vi "Reduce Vitrek Results.vi"(0 "Results String":string, 1 "BW1 ACW Time":string[](array[string]), 2 "BW1 ACW Raw":string[](array[string]), 3 "BW2 ACW Time":string[](array[string]), 4 "BW2 ACW Raw":string[](array[string]), 5 "error in (no error)":errorcluster, 6 "Result Error Status":string, 7 "Dielectric Strength Spec (uA)":dbl=50.0 format="%#_13g", 9 "Insulation Resistance Spec (Mohms)":dbl=100.0 format="%#_13g") -> (11 "BW1 Results Indicator":T1, 13 "BW2 Results Indicator":T1, 14 "Raw Data ACW BW1":T4, 15 "BW 1 Results":T2, 16 "Raw Data ACW BW2":T3, 17 "BW 2 Results":T2, 19 "error out":errorcluster)   [LabVIEW 2018]
panel:
  out "BW2 Insulation Resistance":string
  out "BW1 Insulation Resistance":string
  out "BW2 IR Pass Indicator":u16
  out "BW2 IR Pass?":bool
  out "BW1 IR Pass Indicator":u16
  out "BW1 IR Pass?":bool
  out "BW1 ACW Pass Indicator":u16
  out "BW1 Dielectric Strength Pass?":bool
  out "BW2 Dielectric Strength Pass?":bool
  out "BW2 Max Leakage Current":dbl
  out "BW2 Min Leakage Current":dbl
  out "BW1 Min Leakage Current":dbl
  out "BW1 Max Leakage Current":dbl
  out "BW2 ACW Pass Indicator":u16
  out "BW2 Max Change in Current (A)":dbl
  out "BW1 Max Change in Current (A)":dbl
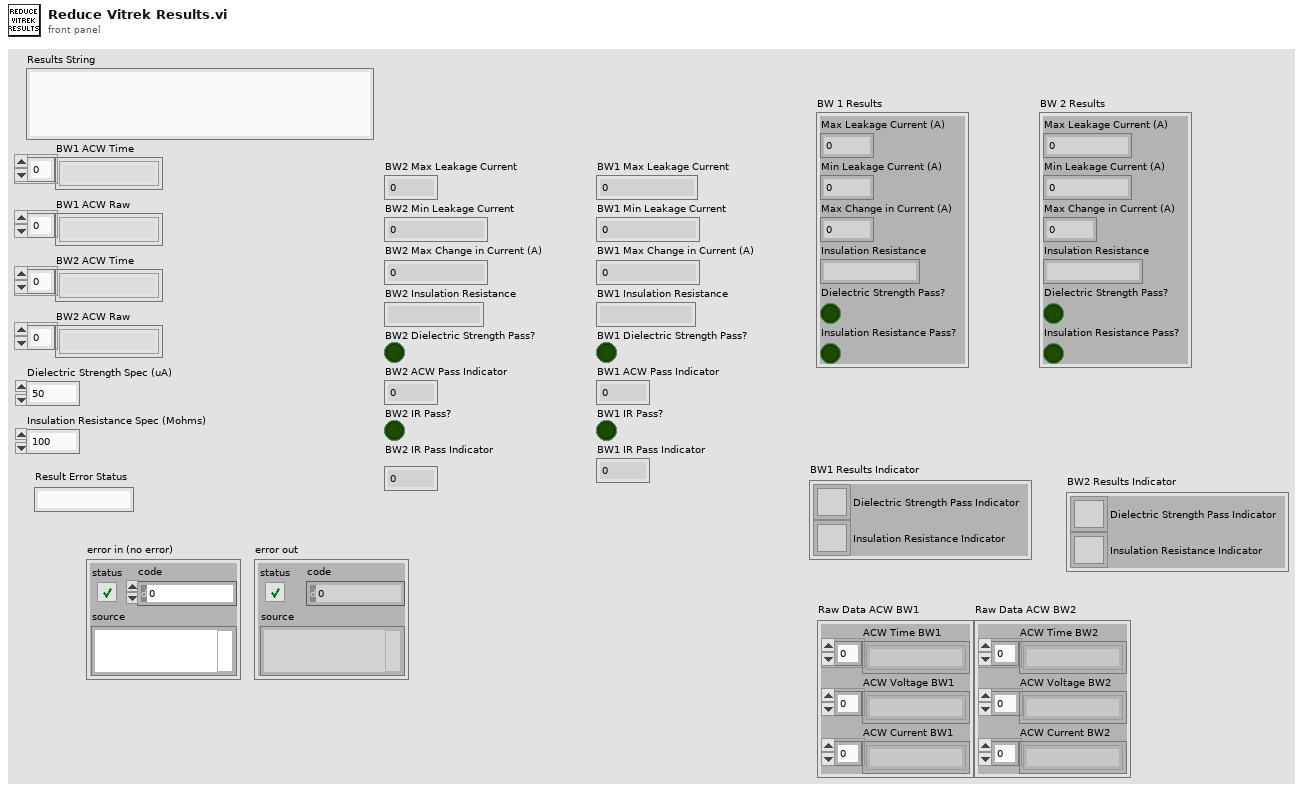
[diagram p1: front panel]
types:
  T1 = cluster{"Dielectric Strength Pass Indicator":u16, "Insulation Resistance Indicator":u16}
  T2 = cluster{"Max Leakage Current (A)":dbl, "Min Leakage Current (A)":dbl, "Max Change in Current (A)":dbl, "Dielectric Strength Pass?":bool, "Insulation Resistance Pass?":bool, "Insulation Resistance":string}
  T3 = cluster{"ACW Time BW2":string[], "ACW Voltage BW2":string[], "ACW Current BW2":string[]}
  T4 = cluster{"ACW Time BW1":string[], "ACW Voltage BW1":string[], "ACW Current BW1":string[]}
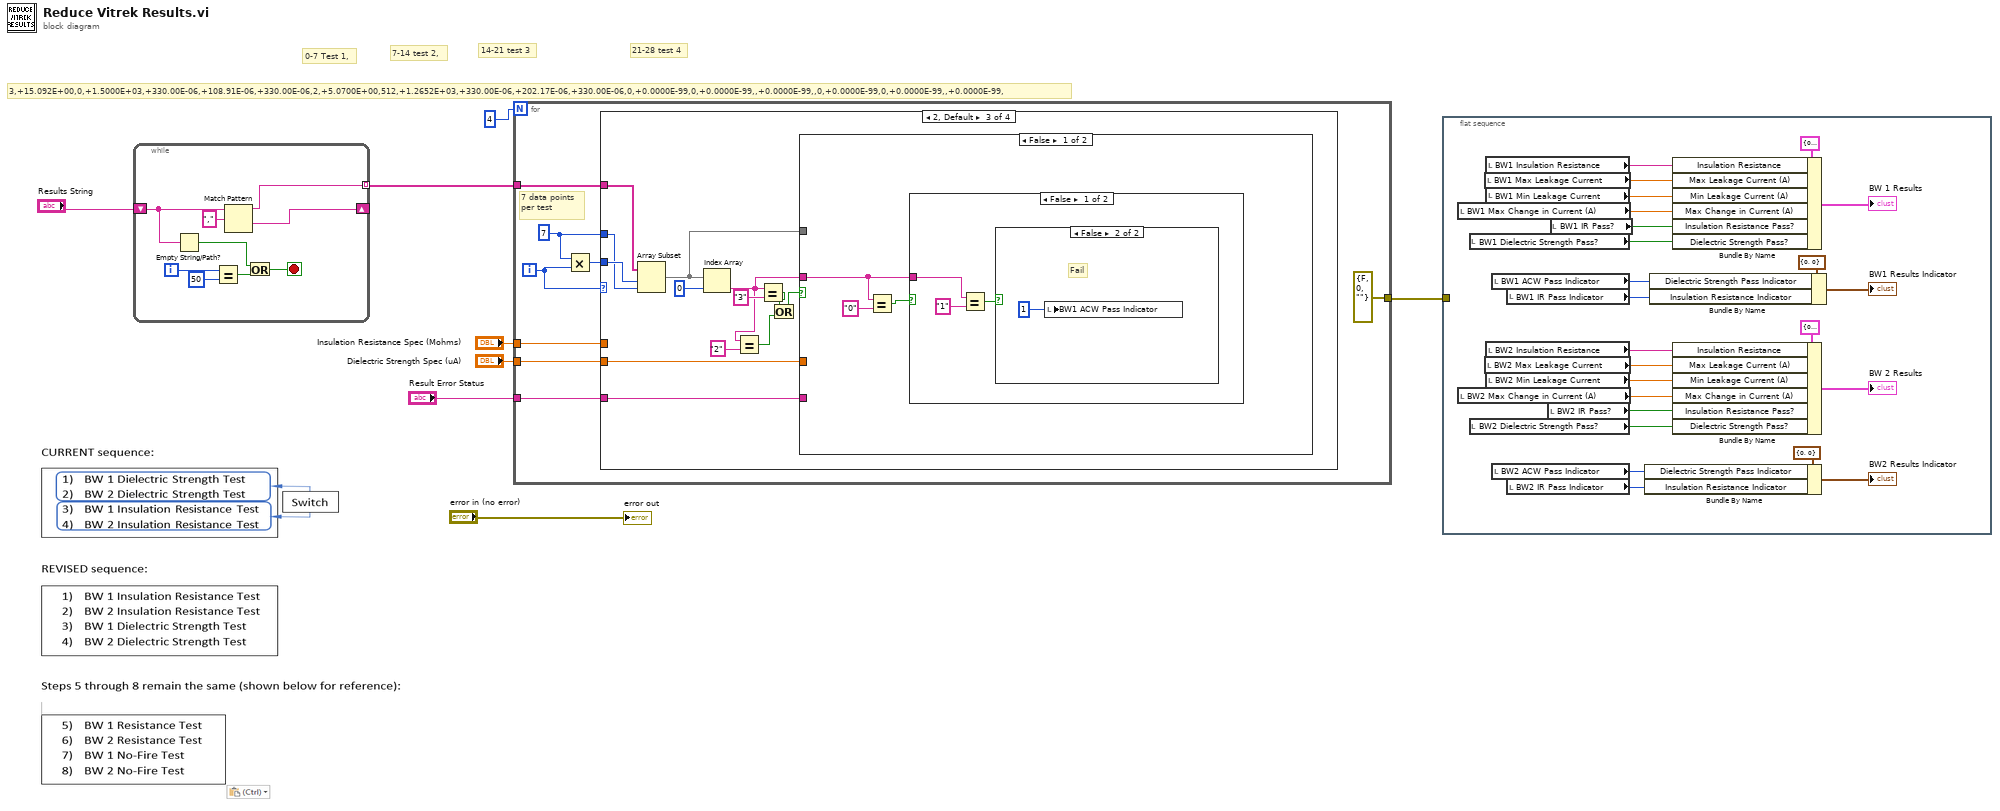
[diagram p0: block diagram]
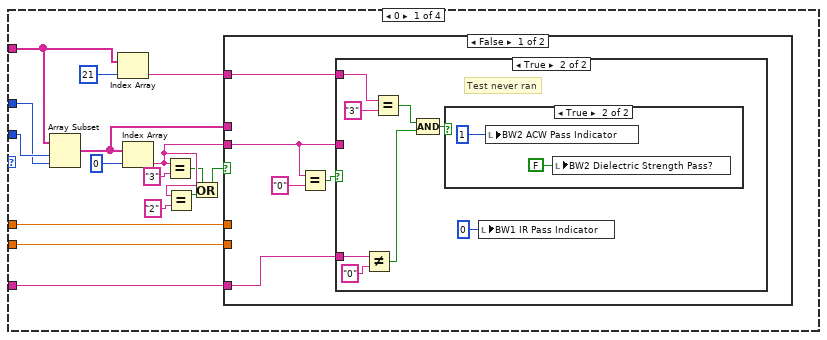
[diagram p2: hidden frame]
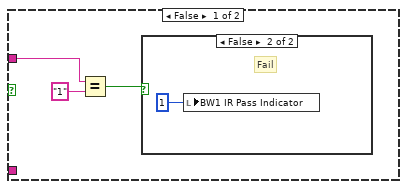
[diagram p3: hidden frame]
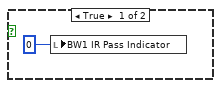
[diagram p4: hidden frame]
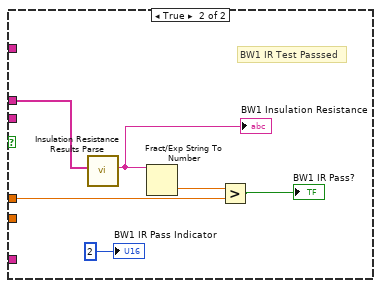
[diagram p6: hidden frame]
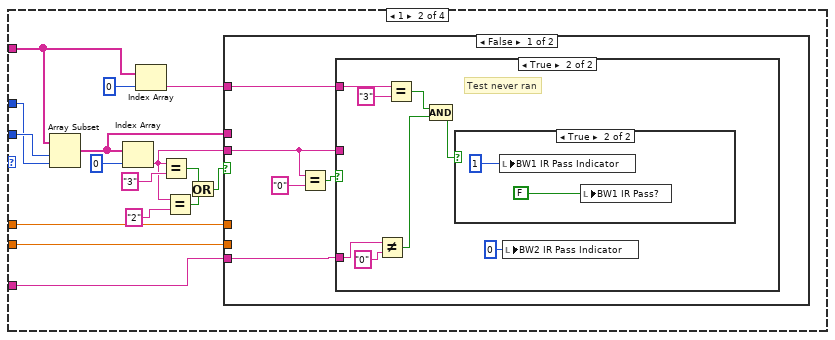
[diagram p7: hidden frame]
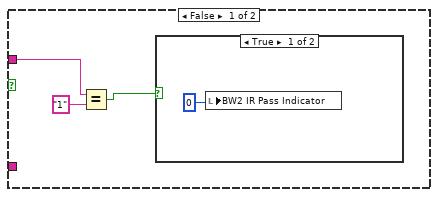
[diagram p8: hidden frame]
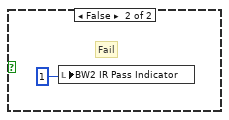
[diagram p9: hidden frame]
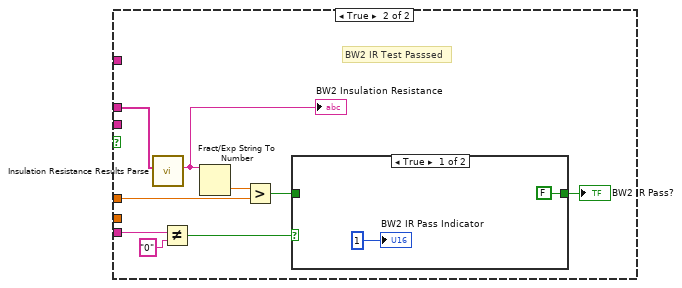
[diagram p11: hidden frame]
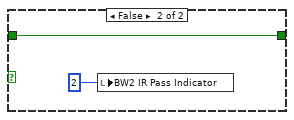
[diagram p12: hidden frame]
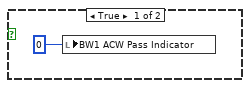
[diagram p13: hidden frame]
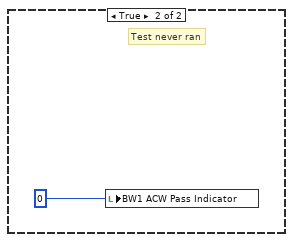
[diagram p14: hidden frame]
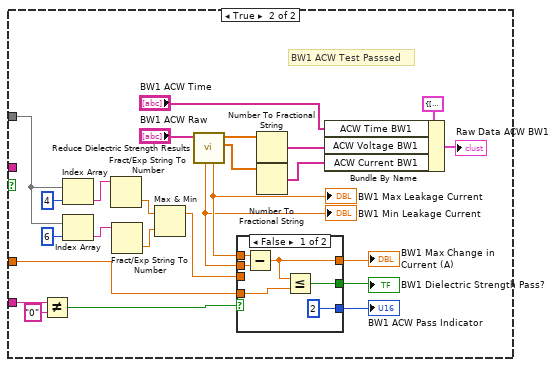
[diagram p15: hidden frame]
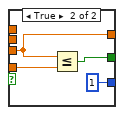
[diagram p16: hidden frame]
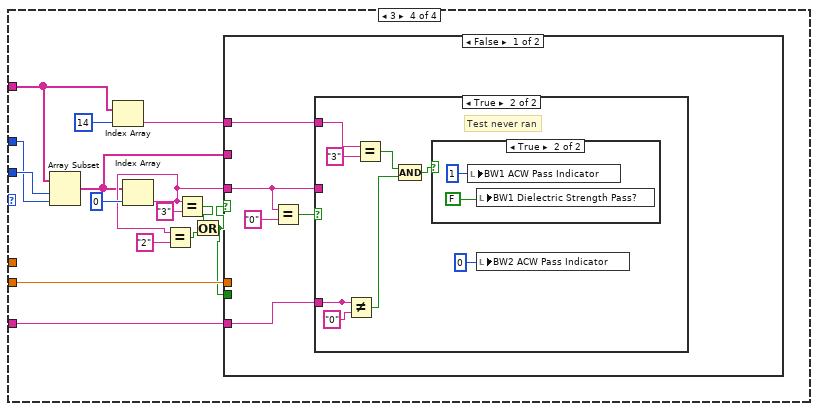
[diagram p17: hidden frame]
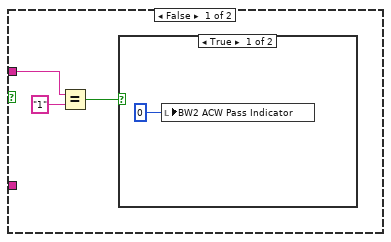
[diagram p18: hidden frame]
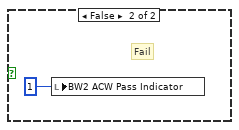
[diagram p19: hidden frame]
diagram:
  # "21-28 test 4"
  # "14-21 test 3"
  # "7-14 test 2,"
  # "0-7 Test 1,"
  # "3,+15.092E+00,0,+1.5000E+03,+330.00E-06,+108.91E-06,+330.00E-06,2,+5.0700E+00,512,+1.2652E+03,+330.00E-06,+202.17E-06,+330.00E-06,0,+0.0000E-99,0,+0.0000E-99,,+0.0000E-99,,0,+0.0000E-99,0,+0.0000E-99,,+0.0000E-99,"
  n1 = while {
    shift-right: [w17] -> _
    shift-left: "Results String" -> [w15]
    tunnel: [w16] -> w6 mode=indexing
    i -> [w13]
    stop <- w9 stop-if-true
    n2 = Empty String/Path?(string/path=w15) -> (empty?=w10:bool)
    n3 = Equal?(x=w13, y=50) -> (x = y?=w11:bool)
    n4 = Match Pattern(string=w15, regular expression=",") -> (before substring=w16:string, after substring=w17:string)  [unwired: 1 in, 2 out]
    n5 = Or(x=w10, y=w11) -> (x .or. y?=w9:bool)
  }
  n6 = for {
    N: 4 -> [_]
    tunnel: w6 -> [w25]
    tunnel: "Dielectric Strength Spec (uA)" -> [w24]
    tunnel: "Insulation Resistance Spec (Mohms)" -> [w23]
    tunnel: [errorcluster {"status"=FALSE, "code"=0, "source"=""} ("error in (no error)")] -> w3
    tunnel: "Result Error Status" -> [w21]
    i -> [w20]
    w18 = 7 ("x")
    # "7 data points\nper test"
    n7 = Multiply(x=w18, y=w20) -> (x*y=w19:i32)
    n8 = case shown="2, Default" w20 {
      tunnel: w25 -> [w35 w77 w127 w184]
      tunnel: w24 -> [w39 w81 w126 w186]
      tunnel: w23 -> [w38 w80 _ _]
      tunnel: w21 -> [w33 w75 w125 w182]
      tunnel: w19 -> [w27 w69 w118 w175]
      tunnel: w18 -> [w26 w68 w117 w174]
      frame 0 {
        n9 = Array Subset(array=w35, index=w27, length=w26) -> (w37:string[])
        n10 = Index Array(array=w35, index=21) -> (element=w34:string)
        n11 = Index Array(array=w37, index=0) -> (element=w31:string)
        n12 = Equal?(x=w31, y="3") -> (x = y?=w29:bool)
        n13 = Equal?(x=w31, y="2") -> (x = y?=w30:bool)
        n14 = Or(x=w29, y=w30) -> (x .or. y?=w28:bool)
        n15 = case shown="False" w28 {
          tunnel: w39 -> [_ _]
          tunnel: w38 -> [_ w64]
          tunnel: w37 -> [_ w62]
          tunnel: w31 -> [w42 _]
          tunnel: w34 -> [w44 _]
          tunnel: w33 -> [w43 _]
          frame False {
            n16 = Equal?(x=w42, y="0") -> (x = y?=w45:bool)
            n17 = case shown="True" w45 {
              tunnel: w44 -> [_ w54]
              tunnel: w43 -> [_ w53]
              tunnel: w42 -> [w48 _]
              frame False {
                n18 = Equal?(x=w48, y="1") -> (x = y?=w47:bool)
                n19 = case shown="False" w47 {
                  frame True {
                    n20 = local write "BW1 IR Pass Indicator"(u16 0 ("BW 1 Resistance Result")) -> ()
                  }
                  frame False {
                    # "Fail"
                    n21 = local write "BW1 IR Pass Indicator"(u16 1 ("BW 1 Resistance Result")) -> ()
                  }
                }
              }
              frame True {
                # "Test never ran"
                n22 = Not Equal?(x=w53, y="0") -> (x != y?=w55:bool)
                n23 = Equal?(x=w54, y="3") -> (x = y?=w57:bool)
                n24 = Compound Arithmetic op=AND(w57, w55) -> (w52:bool)
                n25 = case shown="True" w52 {
                  frame False {
                  }
                  frame True {
                    n26 = local write "BW2 ACW Pass Indicator"(u16 1 ("BW 1 Resistance Result")) -> ()
                    n27 = local write "BW2 Dielectric Strength Pass?"(FALSE ("BW2 Dielectric Strength Pass?")) -> ()
                  }
                }
                n28 = local write "BW1 IR Pass Indicator"(u16 0 ("BW 1 Resistance Result")) -> ()
              }
            }
          }
          frame True {
            # "BW1 IR Test Passsed"
            n29 = call "Insulation Resistance Results Parse.vi"("Insulation Resistance Results In"=w62) -> ("Insulation Resistance"=w66:string)  [unwired: 9 in, 1 out]
            "BW1 Insulation Resistance" <- w66
            n30 = Fract/Exp String To Number(string=w66) -> (number=w65:dbl)  [unwired: 3 in, 1 out]
            n31 = Greater?(x=w65, y=w64) -> (0:→"BW1 IR Pass?":bool)
            "BW1 IR Pass Indicator" <- u16 2 ("BW 1 Resistance Result")
          }
        }
      }
      frame 1 {
        n32 = Array Subset(array=w77, index=w69, length=w68) -> (w79:string[])
        n33 = Index Array(array=w79, index=0) -> (element=w73:string)
        n34 = Index Array(array=w77, index=0) -> (element=w76:string)
        n35 = Equal?(x=w73, y="3") -> (x = y?=w71:bool)
        n36 = Equal?(x=w73, y="2") -> (x = y?=w72:bool)
        n37 = Or(x=w71, y=w72) -> (x .or. y?=w70:bool)
        n38 = case shown="False" w70 {
          tunnel: w81 -> [_ _]
          tunnel: w80 -> [_ w110]
          tunnel: w79 -> [_ w109]
          tunnel: w73 -> [w84 _]
          tunnel: w76 -> [w86 _]
          tunnel: w75 -> [w85 w107]
          frame False {
            n39 = Equal?(x=w84, y="0") -> (x = y?=w87:bool)
            n40 = case shown="True" w87 {
              tunnel: w86 -> [_ w96]
              tunnel: w85 -> [_ w95]
              tunnel: w84 -> [w90 _]
              frame False {
                n41 = Equal?(x=w90, y="1") -> (x = y?=w89:bool)
                n42 = case shown="True" w89 {
                  frame True {
                    n43 = local write "BW2 IR Pass Indicator"(u16 0 ("BW 1 Resistance Result")) -> ()
                  }
                  frame False {
                    # "Fail"
                    n44 = local write "BW2 IR Pass Indicator"(u16 1 ("BW 1 Resistance Result")) -> ()
                  }
                }
              }
              frame True {
                # "Test never ran"
                n45 = Not Equal?(x=w95, y="0") -> (x != y?=w100:bool)
                n46 = Equal?(x=w96, y="3") -> (x = y?=w99:bool)
                n47 = Compound Arithmetic op=AND(w99, w100) -> (w94:bool)
                n48 = case shown="True" w94 {
                  frame False {
                  }
                  frame True {
                    n49 = local write "BW1 IR Pass Indicator"(u16 1 ("BW1 ACW Pass Indicator")) -> ()
                    n50 = local write "BW1 IR Pass?"(FALSE ("BW2 Dielectric Strength Pass?")) -> ()
                  }
                }
                n51 = local write "BW2 IR Pass Indicator"(u16 0 ("BW 1 Resistance Result")) -> ()
              }
            }
          }
          frame True {
            # "BW2 IR Test Passsed"
            n52 = call "Insulation Resistance Results Parse.vi"("Insulation Resistance Results In"=w109) -> ("Insulation Resistance"=w112:string)  [unwired: 9 in, 1 out]
            "BW2 Insulation Resistance" <- w112
            n53 = Not Equal?(x=w107, y="0") -> (x != y?=w106:bool)
            n54 = Fract/Exp String To Number(string=w112) -> (number=w111:dbl)  [unwired: 3 in, 1 out]
            n55 = Greater?(x=w111, y=w110) -> (0:w105:bool)
            n56 = case shown="True" w106 {
              tunnel: w105 -> [_ w115]
              tunnel: [FALSE w115] -> w104
              frame True {
                "BW2 IR Pass Indicator" <- u16 1 ("BW 1 Resistance Result")
              }
              frame False {
                n57 = local write "BW2 IR Pass Indicator"(u16 2 ("BW 1 Resistance Result")) -> ()
              }
            }
            "BW2 IR Pass?" <- w104
          }
        }
      }
      frame 2, Default {
        n58 = Array Subset(array=w127, index=w118, length=w117) -> (w119:string[])
        n59 = Index Array(array=w119, index=0) -> (element=w122:string)
        n60 = Equal?(x=w122, y="2") -> (x = y?=w121:bool)
        n61 = Equal?(x=w122, y="3") -> (x = y?=w124:bool)
        n62 = Or(x=w124, y=w121) -> (x .or. y?=w120:bool)
        n63 = case shown="False" w120 {
          tunnel: w122 -> [w130 _]
          tunnel: w126 -> [_ w145]
          tunnel: w125 -> [_ w146]
          tunnel: w119 -> [_ w139]
          frame False {
            n64 = Equal?(x=w130, y="0") -> (x = y?=w131:bool)
            n65 = case shown="False" w131 {
              tunnel: w130 -> [w134 _]
              frame False {
                n66 = Equal?(x=w134, y="1") -> (x = y?=w133:bool)
                n67 = case shown="False" w133 {
                  frame True {
                    n68 = local write "BW1 ACW Pass Indicator"(u16 0 ("BW 1 Resistance Result")) -> ()
                  }
                  frame False {
                    # "Fail"
                    n69 = local write "BW1 ACW Pass Indicator"(u16 1 ("BW 1 Resistance Result")) -> ()
                  }
                }
              }
              frame True {
                # "Test never ran"
                n70 = local write "BW1 ACW Pass Indicator"(u16 0 ("BW 1 Resistance Result")) -> ()
              }
            }
          }
          frame True {
            # "BW1 ACW Test Passsed"
            n71 = Not Equal?(x=w146, y="0") -> (x != y?=w154:bool)
            n72 = Index Array(array=w139, index=4) -> (element=w150:string)
            n73 = Index Array(array=w139, index=6) -> (element=w149:string)
            n74 = Fract/Exp String To Number(string=w150) -> (number=w148:dbl)  [unwired: 3 in, 1 out]
            n75 = Fract/Exp String To Number(string=w149) -> (number=w147:dbl)  [unwired: 3 in, 1 out]
            n76 = Max & Min(x=w148, y=w147) -> (max(x,y)=w155:dbl)  [unwired: 1 out]
            n77 = call "Reduce Dielectric Strength Results.vi"("Results Array In"="BW1 ACW Raw") -> ("ACW Current"=w160:dbl[], "ACW Voltage"=w159:dbl[], "Max Leakage Current"=w141:dbl, "Min Leakage Current"=w140:dbl)  [unwired: 5 in, 2 out]
            "BW1 Max Leakage Current" <- w141
            "BW1 Min Leakage Current" <- w140
            n78 = case shown="False" w154 {
              tunnel: [w169 w173] -> w144
              tunnel: w140 -> [w168 _]
              tunnel: w141 -> [w167 _]
              tunnel: [w166 w172] -> w143
              tunnel: w155 -> [_ w173]
              tunnel: [u16 2 ("BW 1 Resistance Result") u16 1 ("BW 1 Resistance Result")] -> w142
              tunnel: w145 -> [w164 w170]
              frame False {
                n79 = Subtract(x=w167, y=w168) -> (x-y=w169:dbl)
                n80 = Less Or Equal?(x=w169, y=w164) -> (x <= y?=w166:bool)
              }
              frame True {
                n81 = Less Or Equal?(x=w173, y=w170) -> (x <= y?=w172:bool)
              }
            }
            "BW1 Max Change in Current (A)" <- w144
            "BW1 ACW Pass Indicator" <- w142
            "BW1 Dielectric Strength Pass?" <- w143
            n82 = Number To Fractional String(number=w159) -> (F-format string=w161:string[])  [unwired: 3 in]
            n83 = Number To Fractional String(number=w160) -> (F-format string=w162:string[])  [unwired: 3 in]
            n84 = Bundle By Name(cluster=T4 {"ACW Time BW1"=[], "ACW Voltage BW1"=[], "ACW Current BW1"=[]} ("Raw Data ACW BW1"), "ACW Time BW1"="BW1 ACW Time", "ACW Voltage BW1"=w161, "ACW Current BW1"=w162) -> (→"Raw Data ACW BW1":T4)
          }
        }
      }
      frame 3 {
        n85 = Array Subset(array=w184, index=w175, length=w174) -> (w177:string[])
        n86 = Index Array(array=w184, index=14) -> (element=w183:string)
        n87 = Index Array(array=w177, index=0) -> (element=w178:string)
        n88 = Equal?(x=w178, y="2") -> (x = y?=w180:bool)
        n89 = Equal?(x=w178, y="3") -> (x = y?=w179:bool)
        n90 = Or(x=w179, y=w180) -> (x .or. y?=w176:bool)
        n91 = case shown="False" w176 {
          tunnel: w178 -> [w189 _]
          tunnel: w186 -> [_ w228]
          tunnel: w183 -> [w191 _]
          tunnel: w182 -> [w190 w224]
          tunnel: w177 -> [_ w222]
          tunnel: w176 -> [_ _]
          frame False {
            n92 = Equal?(x=w189, y="0") -> (x = y?=w192:bool)
            n93 = case shown="True" w192 {
              tunnel: w191 -> [_ w200]
              tunnel: w190 -> [_ w199]
              tunnel: w189 -> [w195 _]
              frame False {
                n94 = Equal?(x=w195, y="1") -> (x = y?=w194:bool)
                n95 = case shown="True" w194 {
                  frame True {
                    n96 = local write "BW2 ACW Pass Indicator"(u16 0 ("BW 1 Resistance Result")) -> ()
                  }
                  frame False {
                    # "Fail"
                    n97 = local write "BW2 ACW Pass Indicator"(u16 1 ("BW 1 Resistance Result")) -> ()
                  }
                }
              }
              frame True {
                # "Test never ran"
                n98 = Not Equal?(x=w199, y="0") -> (x != y?=w204:bool)
                n99 = Not Equal?(x=w199, y="0") -> (x != y?=w206:bool)
                n100 = Equal?(x=w200, y="3") -> (x = y?=w202:bool)
                n101 = Equal?(x=w200, y="3") -> (x = y?=w208:bool)
                n102 = Compound Arithmetic op=AND(w202, w204) -> ()  [unwired: 1 out]
                n103 = Compound Arithmetic op=AND(w208, w206) -> (w205:bool)
                n104 = case shown="True" w205 {
                  frame False {
                  }
                  frame True {
                    n105 = local write "BW1 ACW Pass Indicator"(u16 1 ("BW1 ACW Pass Indicator")) -> ()
                    n106 = local write "BW1 Dielectric Strength Pass?"(FALSE ("BW1 IR Pass?")) -> ()
                  }
                }
                n107 = local write "BW2 ACW Pass Indicator"(u16 0 ("BW 1 Resistance Result")) -> ()
              }
            }
          }
          frame True {
            # "BW2 ACW Test Passsed"
            n108 = Not Equal?(x=w224, y="0") -> (x != y?=w215:bool)
            n109 = Index Array(array=w222, index=4) -> (element=w219:string)
            n110 = Index Array(array=w222, index=6) -> (element=w218:string)
            n111 = Fract/Exp String To Number(string=w219) -> (number=w217:dbl)  [unwired: 3 in, 1 out]
            n112 = Fract/Exp String To Number(string=w218) -> (number=w216:dbl)  [unwired: 3 in, 1 out]
            n113 = Max & Min(x=w217, y=w216) -> (max(x,y)=w214:dbl)  [unwired: 1 out]
            n114 = call "Reduce Dielectric Strength Results.vi"("Results Array In"="BW2 ACW Raw") -> ("ACW Current"=w234:dbl[], "ACW Voltage"=w233:dbl[], "Max Leakage Current"=w226:dbl, "Min Leakage Current"=w227:dbl)  [unwired: 5 in, 2 out]
            "BW2 Max Leakage Current" <- w226
            "BW2 Min Leakage Current" <- w227
            n115 = case shown="True" w215 {
              tunnel: [w243 w247] -> w230
              tunnel: w228 -> [w242 w246]
              tunnel: w227 -> [w241 _]
              tunnel: w226 -> [w240 _]
              tunnel: [w239 w245] -> w225
              tunnel: w214 -> [_ w247]
              tunnel: [u16 2 ("BW 1 Resistance Result") u16 1 ("BW 1 Resistance Result")] -> w213
              frame False {
                n116 = Subtract(x=w240, y=w241) -> (x-y=w243:dbl)
                n117 = Less Or Equal?(x=w243, y=w242) -> (x <= y?=w239:bool)
              }
              frame True {
                n118 = Less Or Equal?(x=w247, y=w246) -> (x <= y?=w245:bool)
              }
            }
            "BW2 Max Change in Current (A)" <- w230
            "BW2 ACW Pass Indicator" <- w213
            "BW2 Dielectric Strength Pass?" <- w225
            n119 = Number To Fractional String(number=w233) -> (F-format string=w235:string[])  [unwired: 3 in]
            n120 = Number To Fractional String(number=w234) -> (F-format string=w237:string[])  [unwired: 3 in]
            n121 = Bundle By Name(cluster=T3 {"ACW Time BW2"=[], "ACW Voltage BW2"=[], "ACW Current BW2"=[]} ("Raw Data ACW BW2"), "ACW Time BW2"="BW2 ACW Time", "ACW Voltage BW2"=w235, "ACW Current BW2"=w237) -> (→"Raw Data ACW BW2":T3)
          }
        }
      }
    }
  }
  n122 = flat-sequence {
    tunnel: w3 -> [_]
    frame #0 {
      n123 = local read "BW1 Max Change in Current (A)"() -> (w268:dbl)
      n124 = local read "BW2 Max Change in Current (A)"() -> (w262:dbl)
      n125 = local read "BW1 Dielectric Strength Pass?"() -> (w266:bool)
      n126 = local read "BW2 Dielectric Strength Pass?"() -> (w264:bool)
      n127 = local read "BW1 Max Leakage Current"() -> (w270:dbl)
      n128 = local read "BW2 Max Leakage Current"() -> (w260:dbl)
      n129 = local read "BW1 Insulation Resistance"() -> (w271:string)
      n130 = local read "BW1 Min Leakage Current"() -> (w269:dbl)
      n131 = local read "BW2 Insulation Resistance"() -> (w265:string)
      n132 = local read "BW2 Min Leakage Current"() -> (w261:dbl)
      n133 = local read "BW1 ACW Pass Indicator"() -> (w254:u16)
      n134 = local read "BW2 ACW Pass Indicator"() -> (w248:u16)
      n135 = local read "BW1 IR Pass Indicator"() -> (w253:u16)
      n136 = local read "BW2 IR Pass Indicator"() -> (w249:u16)
      n137 = local read "BW2 IR Pass?"() -> (w263:bool)
      n138 = local read "BW1 IR Pass?"() -> (w267:bool)
      n139 = Bundle By Name(cluster=T1 {"Dielectric Strength Pass Indicator"=0, "Insulation Resistance Indicator"=0} ("BW2 Results Indicator"), "Dielectric Strength Pass Indicator"=w248, "Insulation Resistance Indicator"=w249) -> (→"BW2 Results Indicator":T1)
      n140 = Bundle By Name(cluster=T1 {"Dielectric Strength Pass Indicator"=0, "Insulation Resistance Indicator"=0} ("BW2 Results Indicator"), "Dielectric Strength Pass Indicator"=w254, "Insulation Resistance Indicator"=w253) -> (→"BW1 Results Indicator":T1)
      n141 = Bundle By Name(cluster=T2 {"Max Leakage Current (A)"=0.0, "Min Leakage Current (A)"=0.0, "Max Change in Current (A)"=0.0, "Dielectric Strength Pass?"=FALSE, "Insulation Resistance Pass?"=FALSE, "Insulation Resistance"=""} ("BW 1 Results"), "Insulation Resistance"=w271, "Max Leakage Current (A)"=w270, "Min Leakage Current (A)"=w269, "Max Change in Current (A)"=w268, "Insulation Resistance Pass?"=w267, "Dielectric Strength Pass?"=w266) -> (→"BW 1 Results":T2)
      n142 = Bundle By Name(cluster=T2 {"Max Leakage Current (A)"=0.0, "Min Leakage Current (A)"=0.0, "Max Change in Current (A)"=0.0, "Dielectric Strength Pass?"=FALSE, "Insulation Resistance Pass?"=FALSE, "Insulation Resistance"=""} ("BW 1 Results"), "Insulation Resistance"=w265, "Max Leakage Current (A)"=w260, "Min Leakage Current (A)"=w261, "Max Change in Current (A)"=w262, "Insulation Resistance Pass?"=w263, "Dielectric Strength Pass?"=w264) -> (→"BW 2 Results":T2)
    }
  }
  "error out" <- "error in (no error)"
